vi "Read Next Line.vi"(8 "error in (no error)":errorcluster, 11 "BaseProducer in":refnum<class "BaseProducer.lvclass">) -> (0 "error out":errorcluster, 1 "Operating Point":dbl[](array[numeric]), 2 "Next State":string, 3 "BaseProducer out":refnum<class "BaseProducer.lvclass">)   [LabVIEW 2013, in "BaseProducer.lvclass"]
doc: "This method reads the next line in a file containing colon-delimited states for the combustor system to run through. It then converts the string to an array of floats and stores them for the controller."
uses:
  BaseProducer.lvclass
  BaseProducer.lvclass/BaseProducer.ctl
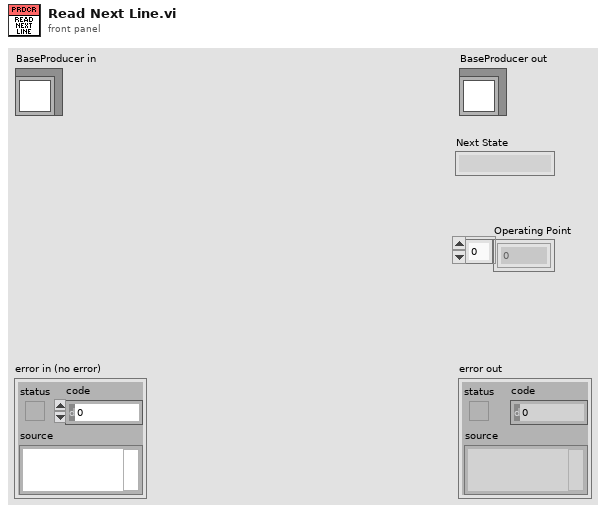
[diagram p1: front panel]
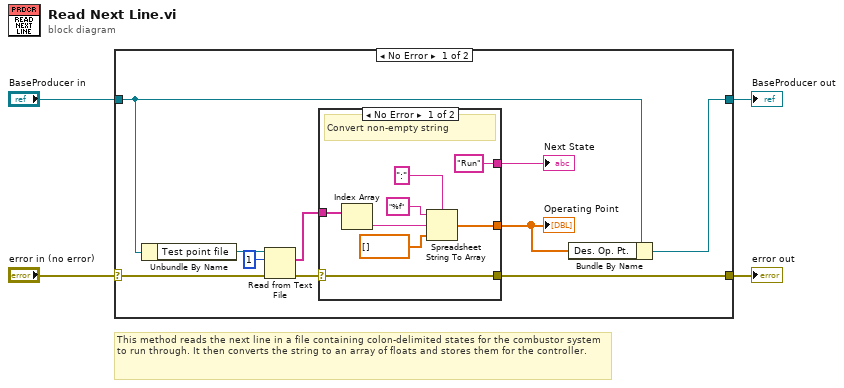
[diagram p0: block diagram]
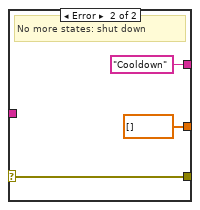
[diagram p2: hidden frame]
diagram:
  # "This method reads the next line in a file containing colon-delimited states for the combustor system to run through. It then converts the string to an array of floats and stores them for the controller."
  n1 = case shown="No Error" "error in (no error)" {
    selector: "error in (no error)" -> [w14 w27]
    tunnel: [w6 w27] -> w3
    tunnel: [w5 w26] -> w1
    tunnel: "BaseProducer in" -> [w9 w26]
    frame No Error {
      n2 = Unbundle By Name(w9) -> ("Test point file"=w13:refnum<file>)
      n3 = Read from Text File(file (use dialog)=w13, count=1, error in=w14) -> (text=w7:string[], error out=w8:errorcluster)  [unwired: 1 in, 2 out]
      n4 = case shown="No Error" w8 {
        selector: w8 -> [w17 w23]
        tunnel: [w17 w23] -> w6
        tunnel: [w19 dbl[] []] -> w11
        tunnel: ["Run" "Cooldown"] -> w10
        tunnel: w7 -> [w16 _]
        frame No Error {
          # "Convert non-empty string"
          n5 = Index Array(array=w16) -> (element=w15:string)  [unwired: 1 in]
          n6 = Spreadsheet String To Array(delimiter (Tab)=":", format string="%f", spreadsheet string=w15, array type (2D Dbl)=dbl[] []) -> (array=w19:dbl[])
        }
        frame Error {
          # "No more states: shut down"
        }
      }
      "Operating Point" <- w11
      "Next State" <- w10
      n7 = Bundle By Name(cluster=w9, "Des. Op. Pt."=w11) -> (w5:refnum<class "BaseProducer.lvclass">)
    }
    frame Error {
    }
  }
  "error out" <- w3
  "BaseProducer out" <- w1
